vi "Read BMP Header Info (excel).vi"(8 "error in (no error)":errorcluster, 11 "BMP file":refnum<file>) -> (0 "error out":errorcluster, 1 "offset to data":u32, 2 "bitmap info":T1, 3 "BMP file":refnum<file>, 4 "color table":u32[](array[colorbox]))   [LabVIEW 2010, in "NI_ReportGenerationToolkit.lvlib"]
doc: "This VI reads in the header information out of a Windows BMP file."
uses:
  <vilib>/addons/_office/NI_ReportGenerationToolkit.lvlib
panel:
  in  "used for datatype only":T1
  in  "uint16":u16
  in  "uint32":u32
  out "file type wrong":bool
  in  "valid depths":u32[](array[numeric])=[1, 4, 8, 24]
  out "bitmap depth is wrong":bool
  out "bitmap is compressed":bool
  out "bitmap header wrong size":bool
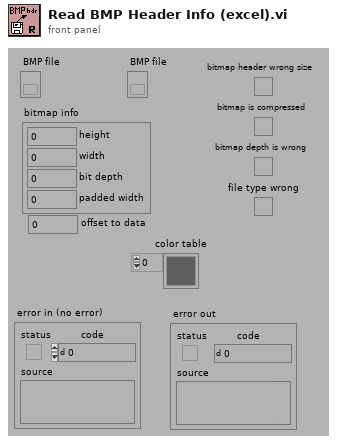
[diagram p1: front panel]
types:
  T1 = cluster{"height":u32, "width":u32, "bit depth":u16, "padded width":u32}
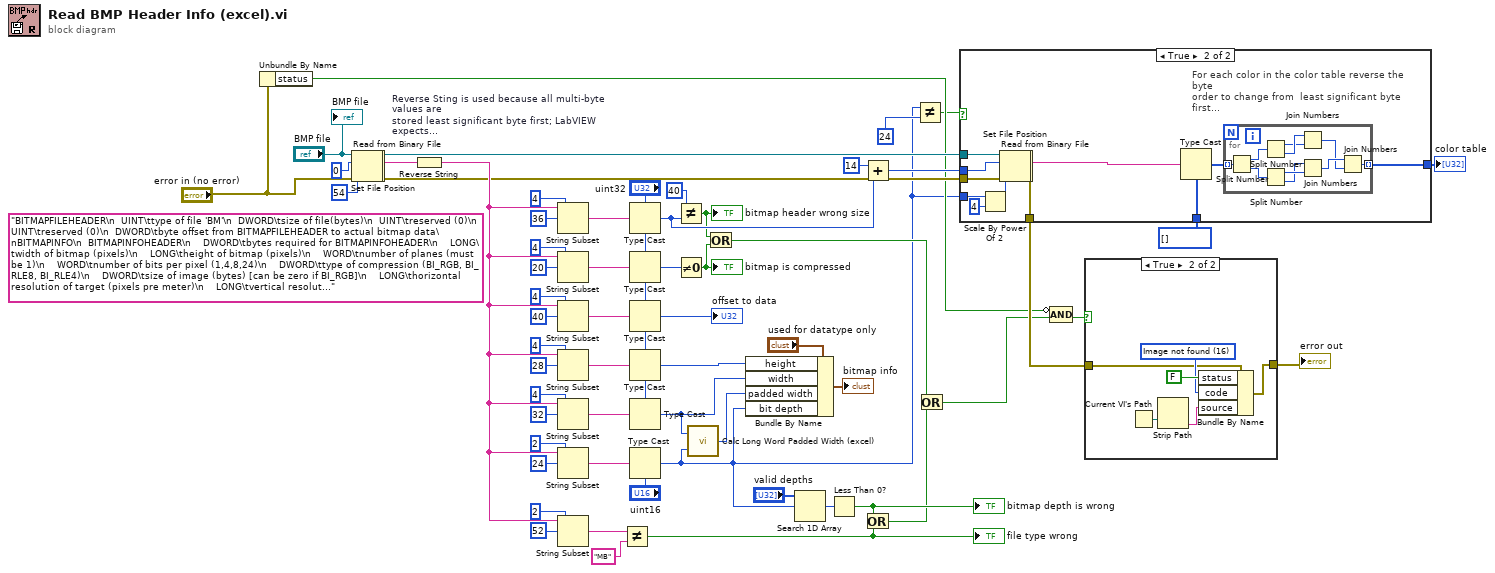
[diagram p0: block diagram]
diagram:
  (unwired) "BITMAPFILEHEADER\n  UINT\ttype of file 'BM'\n  DWORD\tsize of file(bytes)\n  UINT\treserved (0)\n  UINT\treserved (0)\n  DWORD\tbyte offset from BITMAPFILEHEADER to actual bitmap data\nBITMAPINFO\n  BITMAPINFOHEADER\n    DWORD\tbytes required for BITMAPINFOHEADER\n    LONG\twidth of bitmap (pixels)\n    LONG\theight of bitmap (pixels)\n    WORD\tnumber of planes (must be 1)\n    WORD\tnumber of bits per pixel (1,4,8,24)\n    DWORD\ttype of compression (BI_RGB, BI_RLE8, BI_RLE4)\n    DWORD\tsize of image (bytes) [can be zero if BI_RGB]\n    LONG\thorizontal resolution of target (pixels pre meter)\n    LONG\tvertical resolution of target (pixels pre meter)\n    DWORD\tcolors used\n    DWORD\tcolors important\n  RGBQUAD\n    BYTE\tblue\n    BYTE\tgreen\n    BYTE\tred\n    BYTE\treserved (0)"
  n1 = Unbundle By Name("error in (no error)") -> ("status"=w9:bool)
  n2 = Set File Position(offset (in bytes) (0)=0, refnum="BMP file", error in="error in (no error)") -> (refnum out=w2:refnum<file>, error out=w1:errorcluster)  [unwired: 1 out]
  n3 = Read from Binary File(8:w1, 10:54, 11:w2) -> (0:w14:errorcluster, 2:w36:string, 3:w55:refnum<file>)  [unwired: 4 out]
  n4 = Reverse String "Reverse Sting is used because all multi-byte values are\nstored least significant byte first; LabVIEW expects \nmost significant byte first."(1:w36) -> (0:w22:string)
  n5 = String Subset(string=w22, offset (0)=36, length (rest)=4) -> (substring=w21:string)
  n6 = String Subset(string=w22, offset (0)=20, length (rest)=4) -> (substring=w20:string)
  n7 = String Subset(string=w22, offset (0)=40, length (rest)=4) -> (substring=w19:string)
  n8 = String Subset(string=w22, offset (0)=28, length (rest)=4) -> (substring=w18:string)
  n9 = String Subset(string=w22, offset (0)=32, length (rest)=4) -> (substring=w17:string)
  n10 = String Subset(string=w22, offset (0)=24, length (rest)=2) -> (substring=w16:string)
  n11 = String Subset(string=w22, offset (0)=52, length (rest)=2) -> (substring=w26:string)
  n12 = Not Equal?(x=w26, y="MB") -> (x != y?=w34:bool)
  "file type wrong" <- w34
  n13 = Type Cast(type="uint32", x=w21) -> (*(type *) &x=w48:u32)
  n14 = Type Cast(type="uint32", x=w20) -> (*(type *) &x=w45:u32)
  n15 = Type Cast(type="uint32", x=w19) -> (*(type *) &x=→"offset to data":u32)
  n16 = Type Cast(type="uint32", x=w18) -> (*(type *) &x=w29:u32)
  n17 = Type Cast(type="uint32", x=w17) -> (*(type *) &x=w28:u32)
  n18 = Type Cast(type="uint16", x=w16) -> (*(type *) &x=w5:u16)
  n19 = Not Equal?(x=40, y=w48) -> (x != y?=w44:bool)
  "bitmap header wrong size" <- w44
  n20 = Not Equal To 0?(x=w45) -> (x != 0?=w43:bool)
  "bitmap is compressed" <- w43
  n21 = call <vilib>:"Calc Long Word Padded Width (excel).vi"("bit depth"=w5, "width"=w28) -> ("padded width"=w27:i32)
  n22 = Or(x=w44, y=w43) -> (x .or. y?=w42:bool)
  n23 = Bundle By Name(cluster="used for datatype only", "height"=w29, "width"=w28, "padded width"=w27, "bit depth"=w5) -> (→"bitmap info":T1)
  n24 = Search 1D Array(1D array="valid depths", element=w5) -> (index of element=w40:i32)  [unwired: 1 out]
  n25 = Less Than 0?(x=w40) -> (x < 0?=w33:bool)
  "bitmap depth is wrong" <- w33
  n26 = Add(x=14, y=w48) -> (x+y=w49:u32)
  n27 = Or(x=w33, y=w34) -> (x .or. y?=w32:bool)
  n28 = Not Equal?(x=w5, y=24) -> (x != y?=w3:bool)
  n29 = Or(x=w42, y=w32) -> (x .or. y?=w11:bool)
  n30 = case shown="True" w3 {
    tunnel: w55 -> [_ w77]
    tunnel: [w65 w75] -> w54
    tunnel: w49 -> [_ w73]
    tunnel: w14 -> [w64 w72]
    tunnel: [w64 w71] -> w12
    tunnel: u32[] [] ("color table") -> [w65 w70]
    tunnel: w5 -> [_ w69]
    frame False {
    }
    frame True {
      n31 = Scale By Power Of 2(n=w69, x=4) -> (x*2^n=w74:i32)
      n32 = Set File Position(offset (in bytes) (0)=w73, refnum=w77, error in=w72) -> (refnum out=w67:refnum<file>, error out=w66:errorcluster)  [unwired: 1 out]
      n33 = Read from Binary File(8:w66, 10:w74, 11:w67) -> (0:w71:errorcluster, 2:w76:string)  [unwired: 5 out]
      n34 = Type Cast(type=w70, x=w76) -> (*(type *) &x=w68:u32[])
      n35 = for "For each color in the color table reverse the byte\norder to change from  least significant byte first\nto most significant byte first." {
        tunnel: [w88] -> w75 mode=indexing
        tunnel: w68 -> [w79] mode=indexing
        n36 = Split Number(x=w79) -> (hi(x)=w86:u16, lo(x)=w87:u16)
        n37 = Split Number(x=w86) -> (hi(x)=w84:u8, lo(x)=w85:u8)
        n38 = Split Number(x=w87) -> (hi(x)=w83:u8, lo(x)=w82:u8)
        n39 = Join Numbers(hi=w85, lo=w84) -> ((hi.lo)=w80:u16)
        n40 = Join Numbers(hi=w82, lo=w83) -> ((hi.lo)=w81:u16)
        n41 = Join Numbers(hi=w81, lo=w80) -> ((hi.lo)=w88:u32)
      }
    }
  }
  "color table" <- w54
  n42 = Compound Arithmetic op=AND(invert w9, w11) -> (w8:bool)
  n43 = case shown="True" w8 {
    tunnel: [w89 w91] -> w13
    tunnel: w12 -> [w89 w90]
    frame False {
    }
    frame True {
      w94 = u16 16 items=["No error", "Argument error", "Memory is full", "Out of zone", "End of file", "File already open", "Generic file I/O error", "File not found", "File permission error", "Disk is full", "Duplicate path", "Too many files open", "System feature not enabled", "Resource file not found", "Cannot add resource", "Resource not found", "Image not found", "Image memory error", "Pen does not exist", "Config type invalid", "Config token not found", "Config parse error", "Config memory error", "Bad external code format", "Bad external code offset", "External code not present", "Null window", "Destroy window error", "Null menu", "Print aborted", "Bad print record", "Print driver error", "Windows error during printing", "Memory error during printing", "Print dialog error", "Generic print error", "Invalid device refnum", "Device not found", "Device parameter error", "Device unit error", "Cannot open device", "Device call aborted", "Generic error", "Cancelled by user", "Object ID too low", "Object ID too high", "Object not in heap", "Unknown heap", "Unknown object (invalid DefProc)", "Unknown object (DefProc not in table)", "Message out of range", "Invalid (null) method", "Unknown message", "Manager call not supported", "Bad address", "Network operation in progress", "Network operation timed out", "Connection is busy", "Network attribute not supported", "Network error", "Address in use", "System out of memory", "Connection aborted", "Connection refused", "Not connected", "Already connected", "Connection closed", "Initialization error (interapplication manager)", "Bad occurrence", "Wait on unbound occurrence handler", "Occurrence queue overflow", "Datalog type conflict", "Unused", "Unrecognized type (interapplication manager)", "Memory corrupt", "Failed to make temporary DLL", "Old CIN version", "Drag socket not found", "Failed to load drop-object", "Failed to register OLE object", "Failed to release OLE object", "Format specifier type mismatch", "Unknown format specifier", "Too few format specifiers", "Too many format specifiers", "Scan failed", "Newer CIN version", "OLE Convert", "Runtime menu error", "Password tampered", "Unknown error code"]
      n44 = Current VI's Path() -> (path=w92:path)
      n45 = Strip Path(path=w92) -> (name=w93:string)  [unwired: 1 out]
      n46 = Bundle By Name(cluster=w90, "status"=FALSE, "code"=w94, "source"=w93) -> (w91:errorcluster)
    }
  }
  "error out" <- w13
  "BMP file" <- "BMP file"
